vi "generate_question.vi"() -> (3 "Question":dbl)   [LabVIEW 2014]
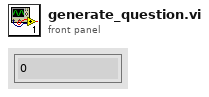
[diagram p1: front panel]
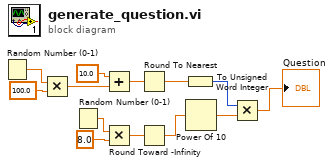
[diagram p0: block diagram]
diagram:
  n1 = Random Number (0-1)() -> (number: 0 to 1=w13:dbl)
  n2 = Multiply(x=w13, y=100.0) -> (x*y=w4:dbl)
  n3 = Random Number (0-1)() -> (number: 0 to 1=w11:dbl)
  n4 = Add(x=10.0, y=w4) -> (x+y=w2:dbl)
  n5 = Multiply(x=w11, y=8.0) -> (x*y=w9:dbl)
  n6 = Round To Nearest(number=w2) -> (nearest integer value=w1:dbl)
  n7 = Round Toward -Infinity(1:w9) -> (0:w8:dbl)
  n8 = To Unsigned Word Integer(number=w1) -> (unsigned 16bit integer=w6:u16)
  n9 = Power Of 10(x=w8) -> (10^x=w7:dbl)
  n10 = Multiply(x=w6, y=w7) -> (x*y=→"Question":dbl)
